vi "CONEX-ALL Reset Controller v2.vi"(9 "Connection Cluster in":T1) -> (3 "Connection Cluster out":T1)   [LabVIEW 2011]
doc: "RS - Reset controller\n\nNo parameters\n\nA 3 second delay is provided to wait for reset."
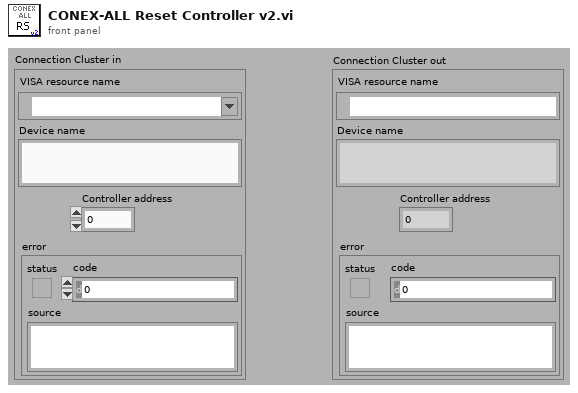
[diagram p1: front panel]
types:
  T1 = cluster{"VISA resource name":refnum<visa-resource-name>, "Device name":string, "Controller address":i32, "error":errorcluster}
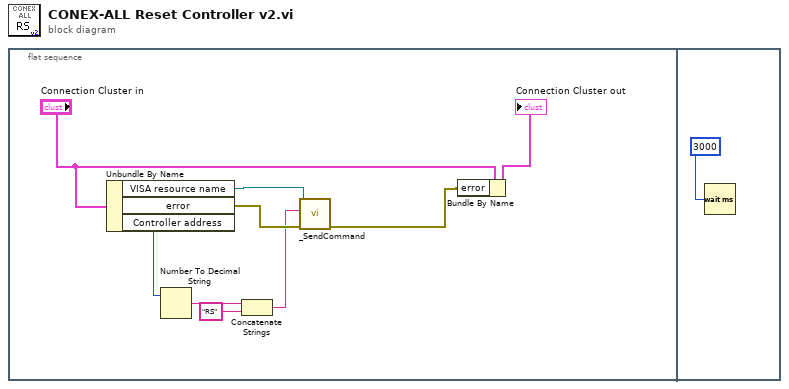
[diagram p0: block diagram]
diagram:
  n1 = flat-sequence {
    frame #0 {
      n2 = Unbundle By Name("Connection Cluster in") -> ("VISA resource name"=w7:refnum<visa-resource-name>, "error"=w5:errorcluster, "Controller address"=w2:i32)
      n3 = Number To Decimal String(number=w2) -> (decimal integer string=w9:string)  [unwired: 1 out]
      n4 = Concatenate Strings(w9, "RS" ("strCommand")) -> (w1:string)
      n5 = call <userlib>:"_SendCommand.vi"("error in"=w5, "Command"=w1, "Instrument Channel"=w7) -> ("error out"=w6:errorcluster)  [unwired: 7 in, 1 out]
      n6 = Bundle By Name(cluster="Connection Cluster in", "error"=w6) -> (→"Connection Cluster out":T1)
    }
    frame #1 {
      n7 = Wait (ms)(milliseconds to wait=3000) -> ()  [unwired: 1 out]
    }
  }
